vi "Process_ManageSemaphore.vi"(4 "error in (no error)":errorcluster, 5 "ms timeout (-1)":i32=-1, 6 "Method (Acquire)":enum8{"Acquire", "Destroy"}(ring), 7 "ref":T1) -> (0 "error out":errorcluster, 2 "Timed out":bool, 3 "semaphore out":T2)   [LabVIEW 2015]
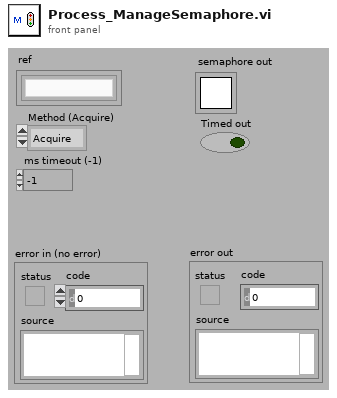
[diagram p1: front panel]
types:
  T1 = typedef "Error站_ref.ctl" = refnum<k1>
  T2 = typedef "Semaphore RefNum" = refnum<k1>
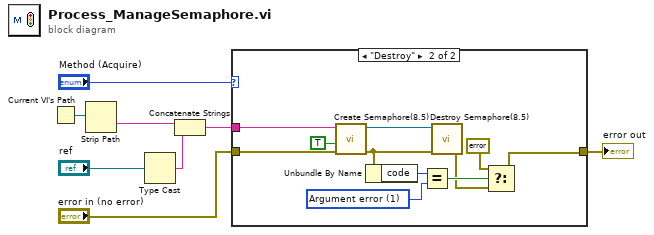
[diagram p0: block diagram]
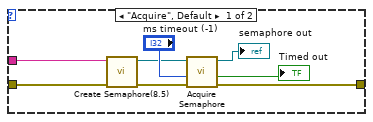
[diagram p2: hidden frame]
diagram:
  n1 = Current VI's Path() -> (path=w6:path)
  n2 = Strip Path(path=w6) -> (name=w4:string)  [unwired: 1 out]
  n3 = Type Cast(x="ref") -> (*(type *) &x=w5:string)  [unwired: 1 in]
  n4 = Concatenate Strings(w4, w5) -> (w8:string)
  n5 = case shown="\"Destroy\"" "Method (Acquire)" {
    tunnel: "error in (no error)" -> [w13 w26]
    tunnel: [w16 w20] -> w2
    tunnel: w8 -> [w14 w27]
    frame "Acquire", Default {
      n6 = call "Create Semaphore(8.5).vi"("error in (no error)"=w13, "name (unnamed)"=w14) -> ("error out"=w10:errorcluster, "semaphore"=w9:T2)  [unwired: 3 in, 1 out]
      n7 = call <vilib>:"Acquire Semaphore.vi"("error in (no error)"=w10, "ms timeout (-1)"="ms timeout (-1)", "semaphore"=w9) -> ("error out"=w16:errorcluster, "timed out"=→"Timed out":bool, "semaphore out"=→"semaphore out":T2)  [unwired: 2 in]
    }
    frame "Destroy" {
      w17 = 1 items=["No error", "Argument error", "Memory is full", "Out of zone", "End of file", "File already open", "Generic file I/O error", "File not found", "File permission error", "Disk is full", "Duplicate path", "Too many files open", "System feature not enabled", "Resource file not found", "Cannot add resource", "Resource not found", "Image not found", "Image memory error", "Pen does not exist", "Config type invalid", "Config token not found", "Config parse error", "Config memory error", "Bad external code format", "Bad external code offset", "External code not present", "Null window", "Destroy window error", "Null menu", "Print aborted", "Bad print record", "Print driver error", "Windows error during printing", "Memory error during printing", "Print dialog error", "Generic print error", "Invalid device refnum", "Device not found", "Device parameter error", "Device unit error", "Cannot open device", "Device call aborted", "Generic error", "Cancelled by user", "Object ID too low", "Object ID too high", "Object not in heap", "Unknown heap", "Unknown object (invalid DefProc)", "Unknown object (DefProc not in table)", "Message out of range", "Invalid (null) method", "Unknown message", "Manager call not supported", "Bad address", "Network operation in progress", "Network operation timed out", "Connection is busy", "Network attribute not supported", "Network error", "Address in use", "System out of memory", "Connection aborted", "Connection refused", "Not connected", "Already connected", "Connection closed", "Initialization error (interapplication manager)", "Bad occurrence", "Wait on unbound occurrence handler", "Occurrence queue overflow", "Datalog type conflict", "Unused", "Unrecognized type (interapplication manager)", "Memory corrupt", "Failed to make temporary DLL", "Old CIN version", "Drag socket not found", "Failed to load drop-object", "Failed to register OLE object", "Failed to release OLE object", "Format specifier type mismatch", "Unknown format specifier", "Too few format specifiers", "Too many format specifiers", "Scan failed", "Newer CIN version", "Error converting to variant", "Runtime menu error", "Password tampered", "Variant attribute not found", "Incompatible variant data type", "Event data is not available", "Event Store is not present", "Occurrence is not found", "Event Queue is not created", "Event info is not available in the type library", "Refnum passed is NULL", "Error retrieving Class GUID", "Error retrieving CoClass GUID", "Error retrieving TypeLib GUID.", "Bad built application magic bytes.", "Specific driver is different from the specific driver associated with the Logical Name.", "There is no session opened to the class driver.", "Max Error", "MAX - Error with config objects", "MAX - Error loading configuration", "MAX - Group not supported", "Singlecast connections can not send to multicast addresses.", "Multicast connections can not send to singlecast addresses.", "Specified IP address not in multicast address range.", "Attempt to write to read-only multicast connection.", "Attempt to read from write-only multicast connection.", "The buffer used to receive a datagram was smaller than the datagram itself"]
      n8 = call "Create Semaphore(8.5).vi"("error in (no error)"=w26, "return existing (F)"=TRUE, "name (unnamed)"=w27) -> ("error out"=w23:errorcluster, "semaphore"=w25:T2)  [unwired: 2 in, 1 out]
      n9 = Unbundle By Name(w23) -> ("code"=w22:i32)
      n10 = Equal?(x=w22, y=w17) -> (x = y?=w21:bool)
      n11 = call "Destroy Semaphore(8.5).vi"("error in (no error)"=w23, "semaphore"=w25) -> ("error out"=w19:errorcluster)  [unwired: 4 in, 1 out]
      n12 = Select(t=errorcluster {"status"=FALSE, "code"=0, "source"=""} ("f"), s=w21, f=w19) -> (s? t:f=w20:errorcluster)
    }
  }
  "error out" <- w2
